vi "Read Header.vi"(7 "Linked List ID":string, 8 "error in (no error)":errorcluster, 10 "Header Name":string, 11 "Linked List Ref":refnum<data-value>) -> (0 "error out":errorcluster, 1 "found":bool, 2 "Header Value":string, 3 "Linked List Ref out":refnum<data-value>)   [LabVIEW 2019, in "Linked Lists.lvlib" / "Linked List Ref.lvclass"]
uses:
  <vilib>/gpm_packages/@cs/linked-list/Source/Linked List/Linked List Ref/Linked List Ref.lvclass
  <vilib>/gpm_packages/@cs/linked-list/Source/Linked List/ILinkedList/ILinked List.lvclass
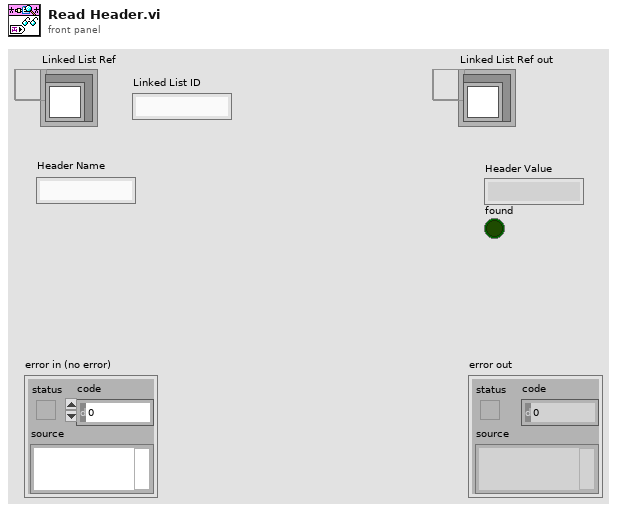
[diagram p1: front panel]
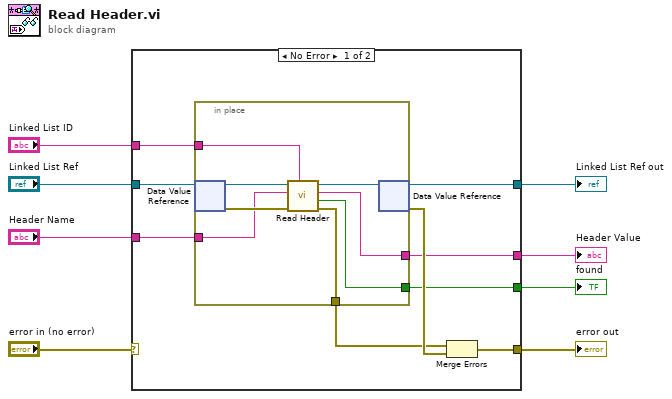
[diagram p0: block diagram]
diagram:
  n1 = case shown="No Error" "error in (no error)" {
    selector: "error in (no error)" -> [_ w27]
    tunnel: "Linked List Ref" -> [w17 w26]
    tunnel: "Linked List ID" -> [w16 _]
    tunnel: "Header Name" -> [w15 _]
    tunnel: [w13 w27] -> w4
    tunnel: [w14 w26] -> w3
    tunnel: [w10 _] -> w1
    tunnel: [w9 _] -> w2
    frame No Error {
      n2 = in-place {
        in-place-border: w16 -> [w24]
        in-place-border: w15 -> [w22]
        in-place-border: [w20] -> w11
        in-place-border: [w19] -> w10
        in-place-border: [w18] -> w9
        n3 = in-place-dvr #1(w17) -> (w25:refnum<class "ILinked List.lvclass">, w23:errorcluster)
        n4 = call-dynamic "Read Header.vi"("Linked List ID"=w24, "error in (no error)"=w23, "Header Name"=w22, "ILinked List in"=w25) -> ("error out"=w20:errorcluster, "found"=w19:bool, "Header Value"=w18:string, "ILinked List out"=w21:refnum<class "ILinked List.lvclass">)  [unwired: 4 in]
        n5 = in-place-dvr #1(w21) -> (w14:refnum<data-value>, w12:errorcluster)
      }
      n6 = Merge Errors(w11, w12) -> (w13:errorcluster)
    }
    frame Error {
    }
  }
  "error out" <- w4
  "Linked List Ref out" <- w3
  "Header Value" <- w2
  "found" <- w1
